vi "findSubject.vi"(8 "error in (no error)":errorcluster, 10 "name":string, 11 "reference in":refnum<class "Subject Controller.lvclass">) -> (0 "error out":errorcluster, 2 "subjectIndex":i32, 3 "reference out":refnum<class "Subject Controller.lvclass">)   [LabVIEW 2015, in "Subject Controller.lvclass"]
uses:
  Subject Controller.lvclass
  APP/subject_class/subject.lvclass
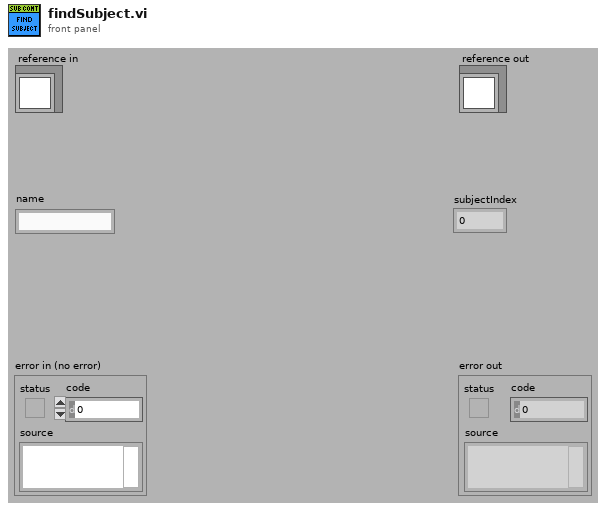
[diagram p1: front panel]
types:
  T1 = typedef "Subject Controller.lvclass/ObjectAttributesRef.ctl" = refnum<data-value>
  T2 = typedef "Subject Controller.lvclass/ObjectAttributes.ctl" = cluster{"MyAttribute":dbl, "subject_controller_ref":refnum<class "Subject Controller.lvclass">, "file_controller_ref":refnum<class "File Controller.lvclass">, "subject_refs":refnum<class "subject.lvclass">[], "subjectIndex":i32, "file_type":T3}
  T3 = typedef "excelFile.lvclass/fileType.ctl" = enum16{"database", "CosmedTest"}
  T4 = cluster{"Ve_warm":dbl[], "time_warm":dbl[], "name":string, "phase":dbl[], "VCO2":dbl[], "VO2":dbl[], "PetCO2":dbl[], "RQ":dbl[], "HR":dbl[], "Ve_warm_inter":dbl[], "time_warm_inter":dbl[], "Ve_exer":dbl[], "time_exer":dbl[], "Ve_exer_inter":dbl[], "time_exer_inter":dbl[], "Ve":dbl[], "time":dbl[]}
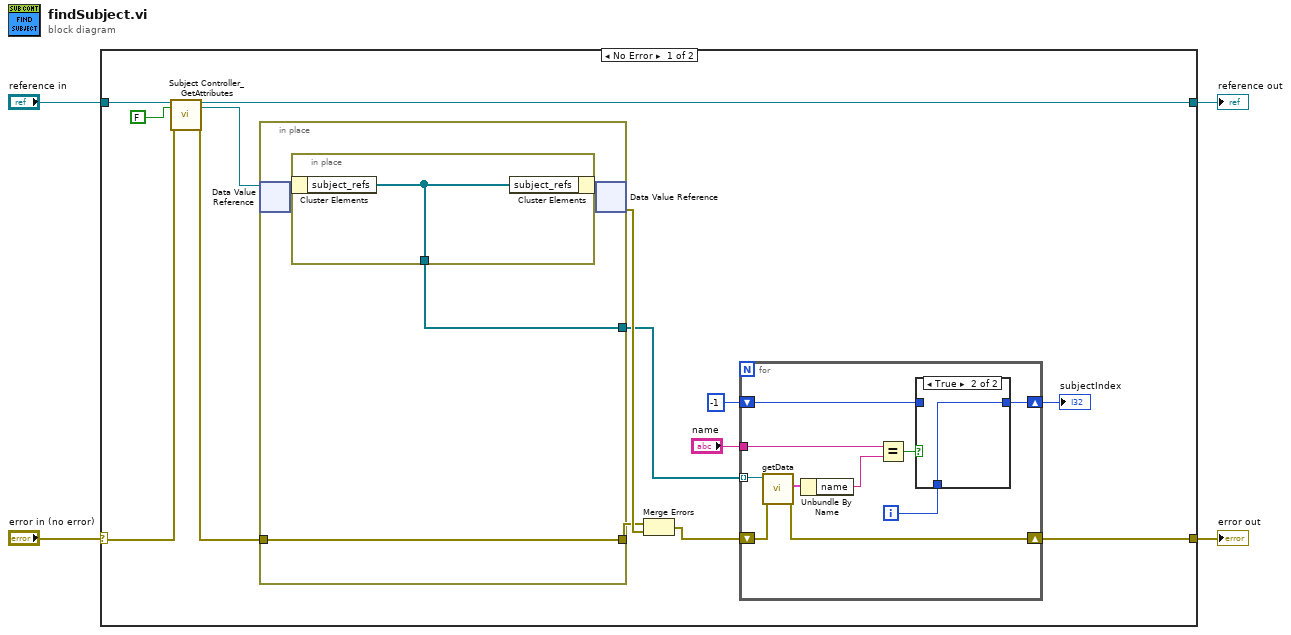
[diagram p0: block diagram]
diagram:
  n1 = case shown="No Error" "error in (no error)" {
    selector: "error in (no error)" -> [w14 w37]
    tunnel: [w8 w37] -> w3
    tunnel: [w12 w36] -> w1
    tunnel: "reference in" -> [w16 w36]
    frame No Error {
      n2 = call "Subject Controller_GetAttributes.vi"("reference in"=w16, "return data? (T)"=FALSE, "error in (no error)"=w14) -> ("reference out"=w12:refnum<class "Subject Controller.lvclass">, "attributes ref"=w11:T1, "error out"=w13:errorcluster)  [unwired: 13 in, 1 out]
      n3 = in-place {
        in-place-border: w13 -> [w32]
        in-place-border: [w32] -> w17
        in-place-border: [w31] -> w10
        n4 = in-place-dvr #1(w11) -> (w33:T2)  [unwired: 1 out]
        n5 = in-place {
          in-place-border: [w35] -> w31
          n6 = in-place-cluster #2(w33) -> ("subject_refs"=w35:refnum<class "subject.lvclass">[])
          n7 = in-place-cluster #2("subject_refs"=w35) -> (w34:T2)
        }
        n8 = in-place-dvr #1(w34) -> (w18:errorcluster)  [unwired: 1 out]
      }
      n9 = Merge Errors(w17, w18) -> (w9:errorcluster)
      n10 = for {
        tunnel: w10 -> [w28] mode=indexing
        tunnel: "name" -> [w25]
        shift-right: [w26] -> w8
        shift-left: w9 -> [w27]
        shift-right: [w21] -> w5
        shift-left: -1 -> [w22]
        i -> [w23]
        n11 = call "getData.vi"("error in (no error)"=w27, "reference in"=w28) -> ("error out"=w26:errorcluster, "data"=w20:T4)  [unwired: 7 in, 1 out]
        n12 = Unbundle By Name(w20) -> ("name"=w19:string)
        n13 = Equal?(x=w25, y=w19) -> (x = y?=w24:bool)
        n14 = case shown="True" w24 {
          tunnel: w23 -> [_ w30]
          tunnel: w22 -> [w29 _]
          tunnel: [w29 w30] -> w21
          frame False {
          }
          frame True {
          }
        }
      }
      "subjectIndex" <- w5
    }
    frame Error {
    }
  }
  "error out" <- w3
  "reference out" <- w1
